vi "Pre Launch Init.vi"(11 "TCPIP Reader in":refnum<class "TCPIP Reader.lvclass">) -> (0 "error out":errorcluster, 3 "TCPIP Reader out":refnum<class "TCPIP Reader.lvclass">)   [LabVIEW 2015, in "TCPIP Reader Actor.lvlib" / "TCPIP Reader.lvclass"]
doc: "(<B>Filename</B>: Actor Framework.lvlib:Actor.lvclass:Pre Launch Init.vi)\n\nDefines behavior that occurs after the Launch Nested Actor method is invoked but before the actor's Actor Core method begins running.\n\nBy default, this method does nothing. A descendant class may override it to define behavior."
uses:
  TCPIP Reader.lvclass
  TCPIP Reader.lvclass/TCPIP Reader.ctl
  <vilib>/ActorFramework/Actor/Actor.lvclass
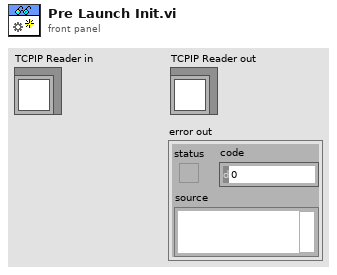
[diagram p1: front panel]
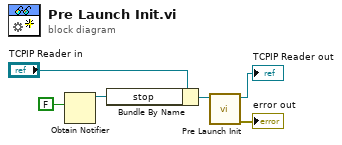
[diagram p0: block diagram]
diagram:
  n1 = Obtain Notifier(notification data type=FALSE) -> (notifier out=w1:refnum<notifier>)  [unwired: 3 in, 2 out]
  n2 = Bundle By Name(cluster="TCPIP Reader in", "stop"=w1) -> (w3:refnum<class "TCPIP Reader.lvclass">)
  n3 = call-parent "Pre Launch Init.vi"("Actor in"=w3) -> ("error out"=→"error out":errorcluster, "Actor out"=→"TCPIP Reader out":refnum<class "TCPIP Reader.lvclass">)  [unwired: 9 in]
